vi "initiate.vi"(8 "error in (no error)":errorcluster, 11 "reference in":refnum<class "PartsTracking Controller.lvclass">) -> (0 "error out":errorcluster, 3 "reference out":refnum<class "PartsTracking Controller.lvclass">)   [LabVIEW 2016, in "PartsTracking Controller.lvclass"]
uses:
  PartsTracking Controller.lvclass
  File Controller_llb/File Controller.lvclass
  GUI/Project Panels_class/Project Panels.lvclass
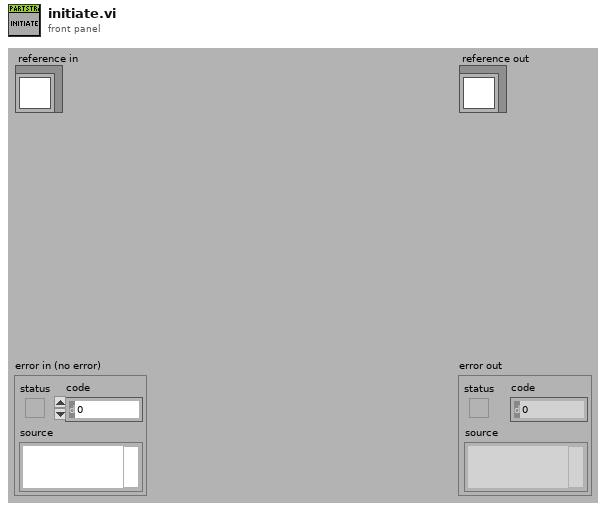
[diagram p1: front panel]
types:
  T1 = typedef "PartsTracking Controller.lvclass/ObjectAttributesRef.ctl" = refnum<data-value>
  T2 = typedef "PartsTracking Controller.lvclass/ObjectAttributes.ctl" = cluster{"MyAttribute":dbl, "file_controller_ref":refnum<class "File Controller.lvclass">, "data":string[][], "partsTracking_ref":refnum<class "partsTracking.lvclass">, "project_panels_ref":refnum<class "Project Panels.lvclass">}
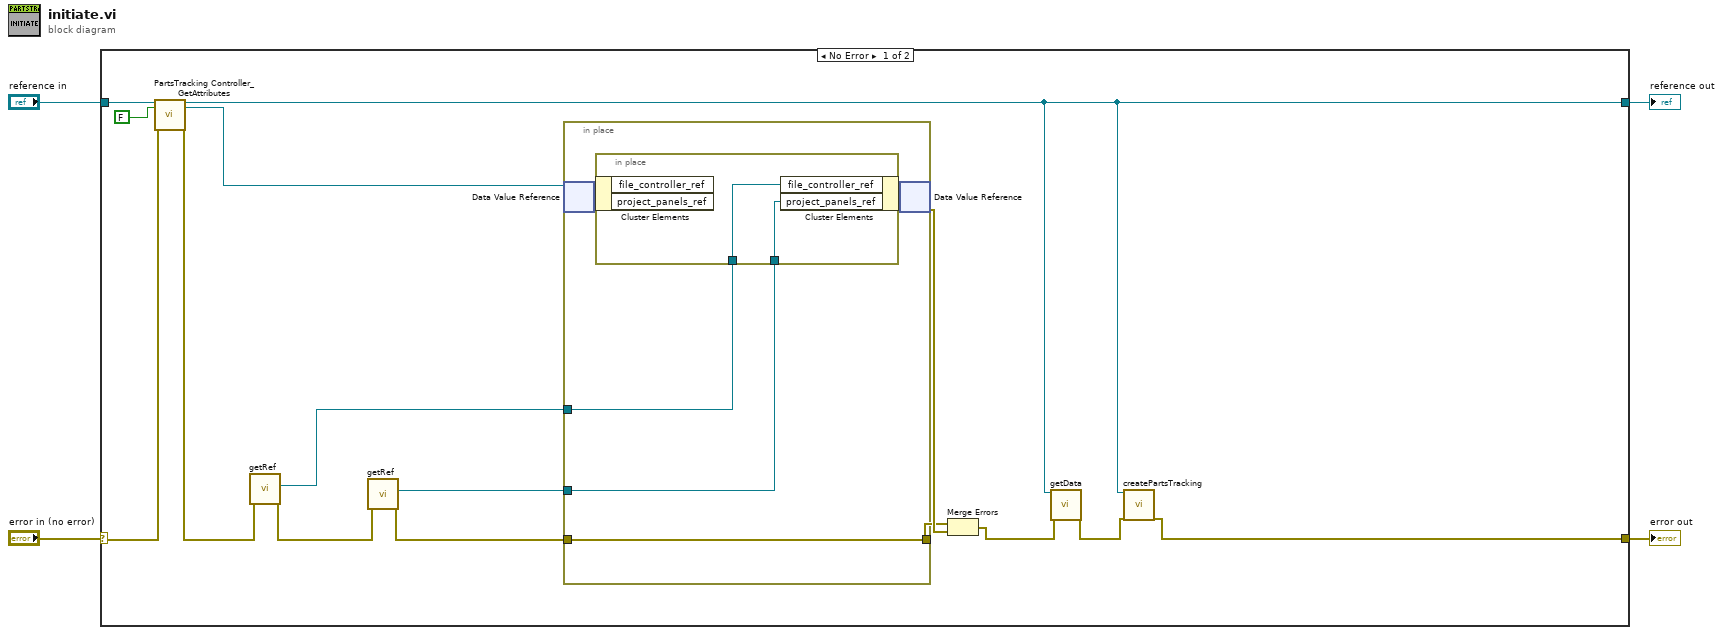
[diagram p0: block diagram]
diagram:
  n1 = case shown="No Error" "error in (no error)" {
    selector: "error in (no error)" -> [w15 w28]
    tunnel: [w8 w28] -> w3
    tunnel: [w10 w27] -> w1
    tunnel: "reference in" -> [w17 w27]
    frame No Error {
      n2 = call "PartsTracking Controller_GetAttributes.vi"("reference in"=w17, "return data? (T)"=FALSE, "error in (no error)"=w15) -> ("reference out"=w10:refnum<class "PartsTracking Controller.lvclass">, "attributes ref"=w14:T1, "error out"=w13:errorcluster)  [unwired: 13 in, 1 out]
      n3 = call "getRef.vi"("error in (no error)"=w13) -> ("error out"=w6:errorcluster, "File Controller_ref"=w12:refnum<class "File Controller.lvclass">)  [unwired: 9 in]
      n4 = call "getRef.vi"("error in (no error)"=w6) -> ("error out"=w5:errorcluster, "project_panels_ref"=w7:refnum<class "Project Panels.lvclass">)  [unwired: 9 in]
      n5 = in-place {
        in-place-border: w5 -> [w22]
        in-place-border: [w22] -> w18
        in-place-border: w12 -> [w21]
        in-place-border: w7 -> [w20]
        n6 = in-place-dvr #1(w14) -> (w23:T2)  [unwired: 1 out]
        n7 = in-place {
          in-place-border: w21 -> [w26]
          in-place-border: w20 -> [w25]
          n8 = in-place-cluster #2(w23) -> ()  [unwired: 2 out]
          n9 = in-place-cluster #2("file_controller_ref"=w26, "project_panels_ref"=w25) -> (w24:T2)
        }
        n10 = in-place-dvr #1(w24) -> (w19:errorcluster)  [unwired: 1 out]
      }
      n11 = Merge Errors(w18, w19) -> (w11:errorcluster)
      n12 = call "getData.vi"("reference in"=w10, "error in (no error)"=w11) -> ("error out"=w9:errorcluster)  [unwired: 16 in, 1 out]
      n13 = call "createPartsTracking.vi"("reference in"=w10, "error in (no error)"=w9) -> ("error out"=w8:errorcluster)  [unwired: 16 in, 1 out]
    }
    frame Error {
    }
  }
  "error out" <- w3
  "reference out" <- w1
